vi "MoveTo.vi"(8 "error in":errorcluster, 11 "Pose":dbl[][](array[numeric])) -> (0 "error out":errorcluster)   [LabVIEW 2013]
uses:
  CRCL Globals.vi
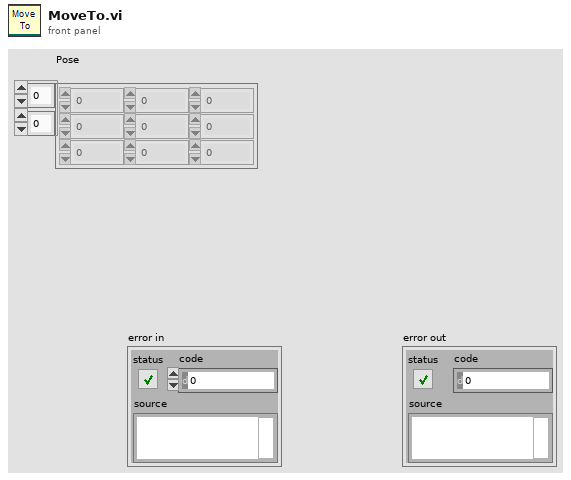
[diagram p1: front panel]
types:
  T1 = typedef "NI_Matrix.lvlib/RealMatrix.ctl" = dbl[][]
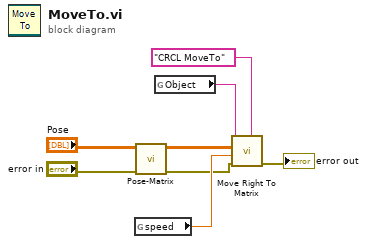
[diagram p0: block diagram]
diagram:
  n1 = global read "CRCL Globals.vi" "speed"() -> (w4:dbl)
  n2 = call "Pose-Matrix.vi"("error in"="error in", "pose"="Pose") -> ("error out"=w3:errorcluster, "T"=w7:T1)  [unwired: 8 in]
  n3 = global read "CRCL Globals.vi" "Object"() -> (w6:string)
  n4 = call "Move Right To Matrix.vi"("Label"="CRCL MoveTo", "error in"=w3, "Speed (mm/s)"=w4, "Goal Pose in Location"=w7, "Location"=w6) -> ("error out"=→"error out":errorcluster)  [unwired: 6 in]
